vi "CR-扫码枪参数读取.vi"(7 "error in (no error)":errorcluster caption="错误输入（无错误）", 10 "基路径":path) -> (0 "error out":errorcluster caption="错误输出", 1 "扫码枪参数":T2={"IsNorImage"=TRUE, "Exposure Values"=100289, "ImagePath"=path "C:/Users/hedongpo/Desktop/514-hdp/Alignment Assemble System/Test Picture/B/3.bmp", "数据输出"="", "结果显示"=FALSE} caption="参数界面" {"Exposure Values" scale=0.0..200000.0}, 2 "扫码枪基础参数":T1 caption="参数界面")   [LabVIEW 2017]
uses:
  <vilib>/Utility/xml.llb/Read From XML File(string).vi
  Global System.vi
panel:
  out "基路径 2":path
  # "UI电源线反面标签1基础参数"
  # "D:\\Inspect System\\Source Code\\Template Program\\BlackTemplete"
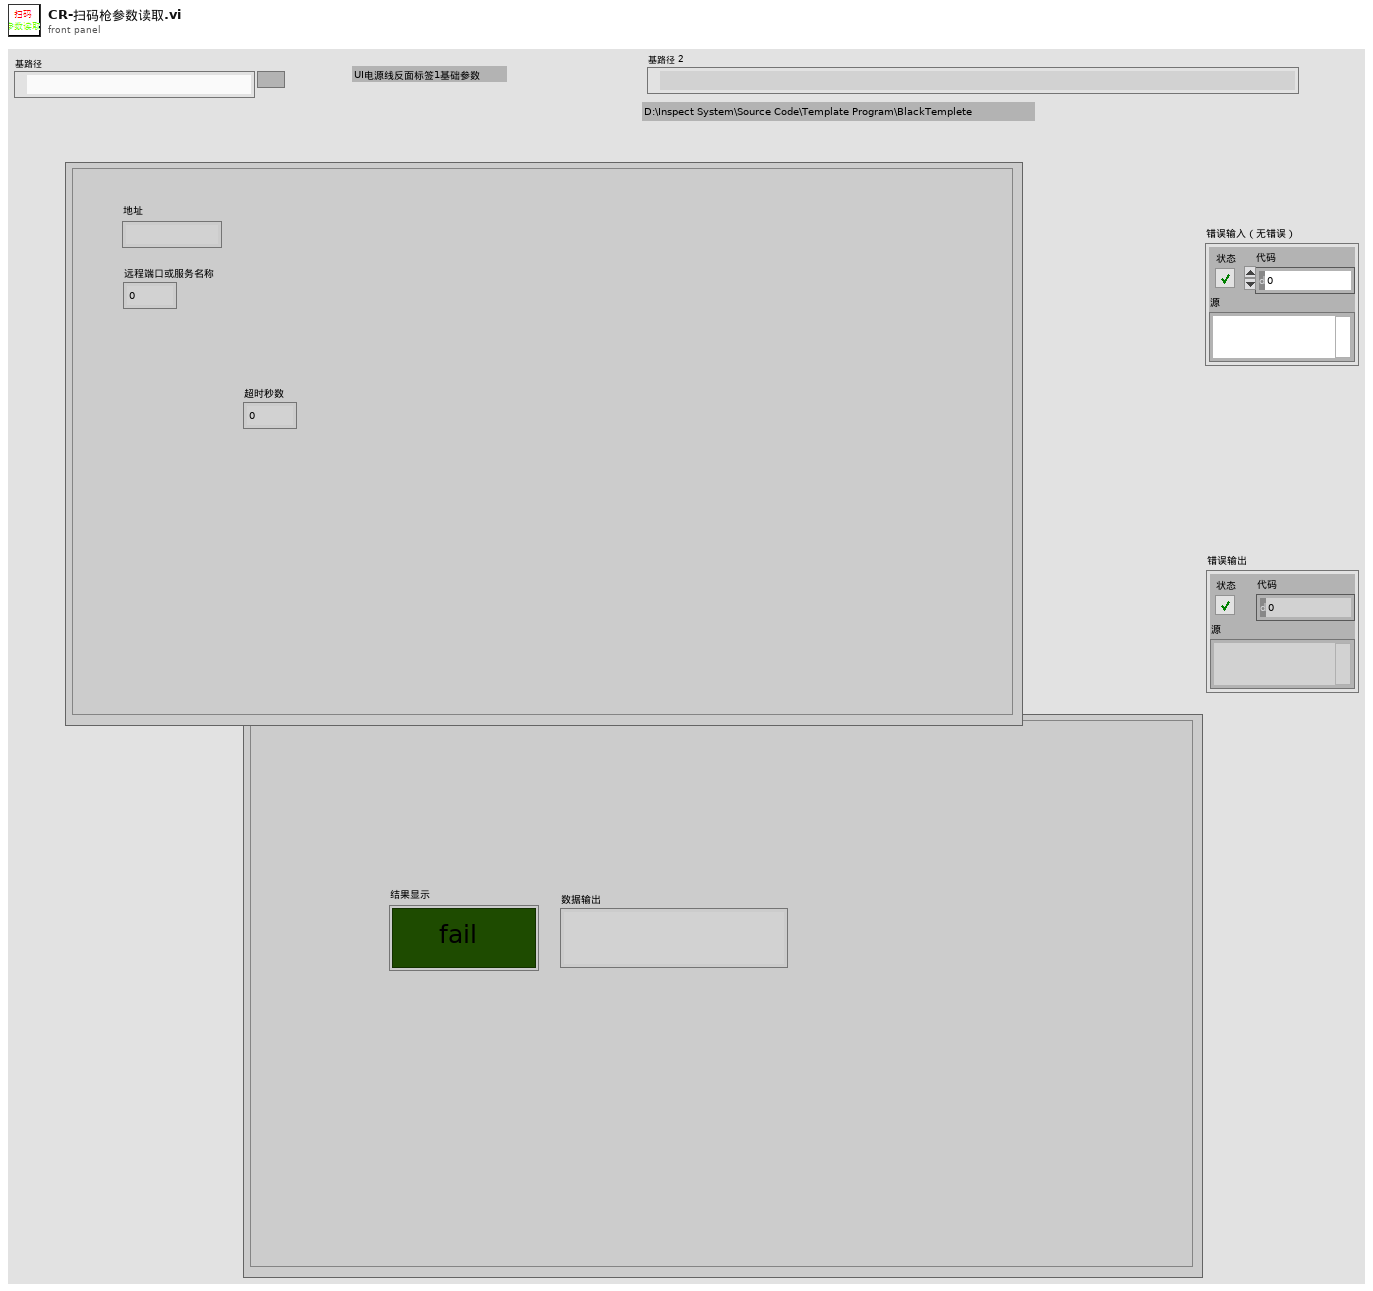
[diagram p1: front panel]
types:
  T1 = cluster{"地址":string, "远程端口或服务名称":u16, "超时秒数":dbl}
  T2 = cluster{"IsNorImage":bool, "Exposure Values":u32, "ImagePath":path, "数据输出":string, "结果显示":bool}
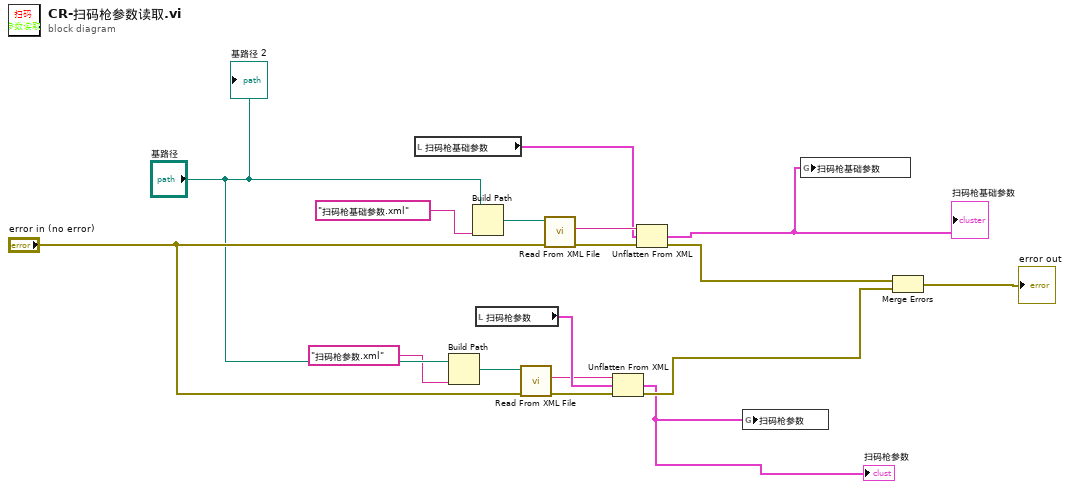
[diagram p0: block diagram]
diagram:
  n1 = local read "扫码枪基础参数"() -> (w14:T1)
  n2 = Build Path(base path="基路径", name or relative path="扫码枪参数.xml" ("名称或相对路径")) -> (appended path=w5:path)
  n3 = Build Path(base path="基路径", name or relative path="扫码枪基础参数.xml" ("名称或相对路径")) -> (appended path=w16:path)
  n4 = local read "扫码枪参数"() -> (w7:T2)
  n5 = call-poly <vilib>:"Read From XML File.vi"("error in (no error)"="error in (no error)", "XML File Path"=w5) -> ("error out"=w4:errorcluster, "XML Elements"=w6:string)  [unwired: 7 in, 1 out]
  n6 = call-poly <vilib>:"Read From XML File.vi"("error in (no error)"="error in (no error)", "XML File Path"=w16) -> ("error out"=w13:errorcluster, "XML Elements"=w15:string)  [unwired: 7 in, 1 out]
  n7 = Unflatten From XML(xml string=w6, type=w7, error in (no error)=w4) -> (value=w2:T2, error out=w11:errorcluster)
  "扫码枪参数" <- w2
  n8 = Unflatten From XML(xml string=w15, type=w14, error in (no error)=w13) -> (value=w1:T1, error out=w12:errorcluster)
  "扫码枪基础参数" <- w1
  n9 = global write "Global System.vi" "扫码枪参数"(w2) -> ()
  n10 = global write "Global System.vi" "扫码枪基础参数"(w1) -> ()
  n11 = Merge Errors(w12, w11) -> (→"error out":errorcluster)
  "基路径 2" <- "基路径"
